vi "Read Configuration.vi"(8 "error in (no error)":errorcluster, 11 "Process In":refnum<class "Process.lvclass">) -> (0 "error out":errorcluster, 3 "Process Out":refnum<class "Process.lvclass">)   [LabVIEW 2020, in "Process.lvclass"]
doc: "Method that read any necessay configurations from config file or potentially configure hard coded values. \nIt is important to set the configured attributes by value and not send commands to the process loop."
uses:
  Process.lvclass
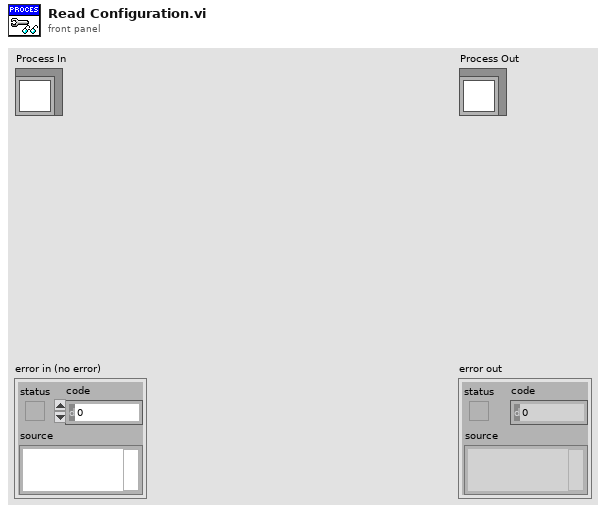
[diagram p1: front panel]
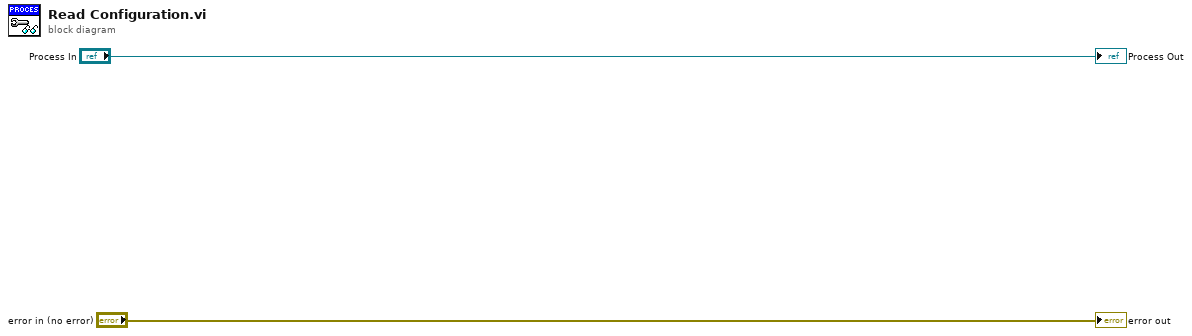
[diagram p0: block diagram]
diagram:
  "error out" <- "error in (no error)"
  "Process Out" <- "Process In"
